vi "MathOptim-Power 2 Estimate.vi"(0 "Y":dbl[](array[numeric]), 5 "X":dbl[](array[numeric])) -> (4 "Initial guess":dbl[](array[numeric]))   [LabVIEW 2020]
uses:
  <vilib>/Analysis/baseanly.llb/Mean (DBL).vi
  Array Manipulation VIs/Irregular Array Subset (DBL).vi
  <vilib>/Analysis/NI_AALBase.lvlib
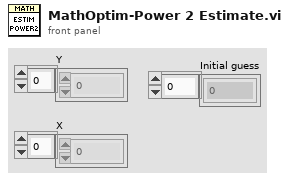
[diagram p1: front panel]
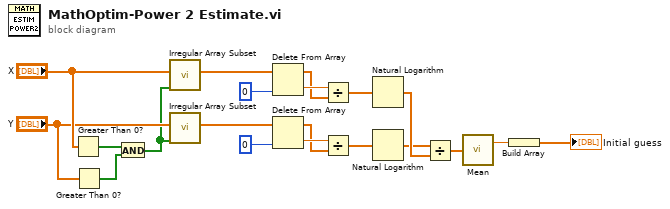
[diagram p0: block diagram]
diagram:
  n1 = Greater Than 0?(x="X") -> (x > 0?=w20:bool[])
  n2 = Greater Than 0?(x="Y") -> (x > 0?=w19:bool[])
  n3 = And(x=w20, y=w19) -> (x .and. y?=w16:bool[])
  n4 = call-poly "Irregular Array Subset.vi"("Mask"=w16, "Array"="X") -> ("Array Subset"=w15:dbl[])  [unwired: 8 in, 1 out]
  n5 = call-poly "Irregular Array Subset.vi"("Mask"=w16, "Array"="Y") -> ("Array Subset"=w6:dbl[])  [unwired: 8 in, 1 out]
  n6 = Delete From Array(array=w15, index=0 ("length")) -> (deleted portion=w13:dbl, array with subset deleted=w12:dbl[])  [unwired: 1 in]
  n7 = Delete From Array(array=w6, index=0 ("length")) -> (deleted portion=w9:dbl, array with subset deleted=w8:dbl[])  [unwired: 1 in]
  n8 = Divide(x=w13, y=w12) -> (x/y=w11:dbl[])
  n9 = Divide(x=w9, y=w8) -> (x/y=w7:dbl[])
  n10 = Natural Logarithm(1:w11) -> (0:w5:dbl[])
  n11 = Natural Logarithm(1:w7) -> (0:w4:dbl[])
  n12 = Divide(x=w4, y=w5) -> (x/y=w3:dbl[])
  n13 = call-poly <vilib>:"Mean.vi"("X"=w3) -> ("mean"=w2:dbl)  [unwired: 1 out]
  n14 = Build Array(w2) -> (→"Initial guess":dbl[])
